vi "Gather Mean.vi"(10 "JSON Scalar":refnum<class "JSON Scalar.lvclass">, 11 "JSON Value In":refnum<class "JSON Value.lvclass">) -> (3 "JSON Statistic or Object":refnum<class "JSON Value.lvclass">)   [LabVIEW 2020, in "Library Commun.lvlib" / "JSON Scalar.lvclass"]
uses:
  JSON Scalar.lvclass
  JSON Value/JSON Value.lvclass
  C:/Users/ngarcin/OneDrive - Altyor/Standard TB/Class/JSON API/JSON Value/JSON Value.lvclass
  JSON Running Mean/JSON Running Mean.lvclass
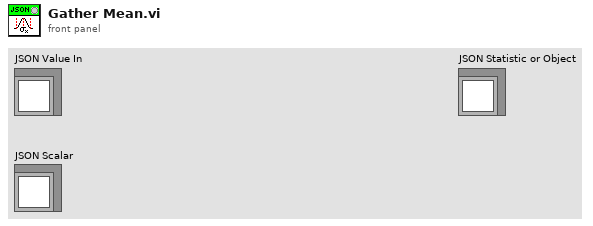
[diagram p1: front panel]
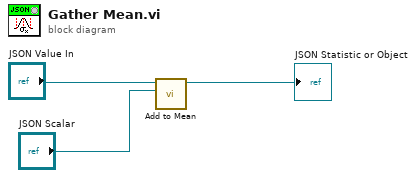
[diagram p0: block diagram]
diagram:
  n1 = call-dynamic "Add to Mean.vi"("Non Object"="JSON Scalar", "JSON Value In"="JSON Value In") -> ("JSON Mean out"=→"JSON Statistic or Object":refnum<class "JSON Running Mean.lvclass">)  [unwired: 9 in]
